vi "Convert Digital Output Level Units.vi"(9 "New output level units":string(combo)="dBFS" caption="SNR", 10 "Previous output level units":string(combo)="dBFS" caption="SNR", 11 "Previous output level":dbl) -> (3 "New output level":dbl)   [LabVIEW 2021]
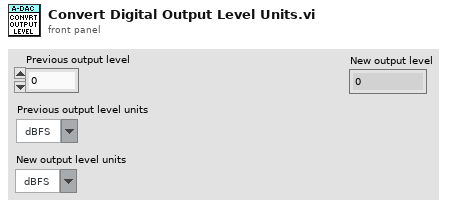
[diagram p1: front panel]
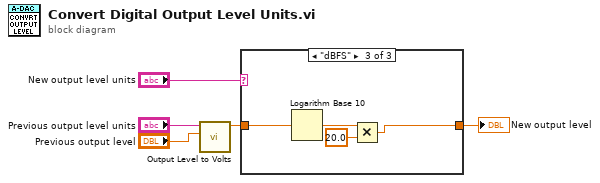
[diagram p0: block diagram]
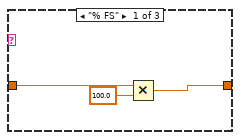
[diagram p2: hidden frame]
diagram:
  n1 = call "Output Level to Volts.vi"("Output level in"="Previous output level", "Output level units"="Previous output level units") -> ("Output level out"=w4:dbl)  [unwired: 9 in]
  n2 = case shown="\"dBFS\"" "New output level units" {
    tunnel: w4 -> [w8 w9 w13]
    tunnel: [w6 w9 w11] -> w3
    frame "% FS" {
      n3 = Multiply(x=w8, y=100.0) -> (x*y=w6:dbl)
    }
    frame "V", Default {
      # "no conversion"
    }
    frame "dBFS" {
      # "convert to desired units"
      n4 = Logarithm Base 10(1:w13) -> (0:w12:dbl)
      n5 = Multiply(x=w12, y=20.0) -> (x*y=w11:dbl)
    }
  }
  "New output level" <- w3
